vi "SUB_TimeGAP_SFCS_RTC.vi"(1 "SFCS year":i32, 2 "UUT_DateTime_input":string="20140703155955", 3 "SFCS month":i32, 4 "SFCS day":i32, 5 "SFCS hour":i32, 6 "SFCS minute":i32, 7 "SFCS second":i32) -> (0 "TimeGap(sec)":dbl format="%#_8f")   [LabVIEW 2011]
panel:
  out "current time":timestamp
  out "time stamp":timestamp
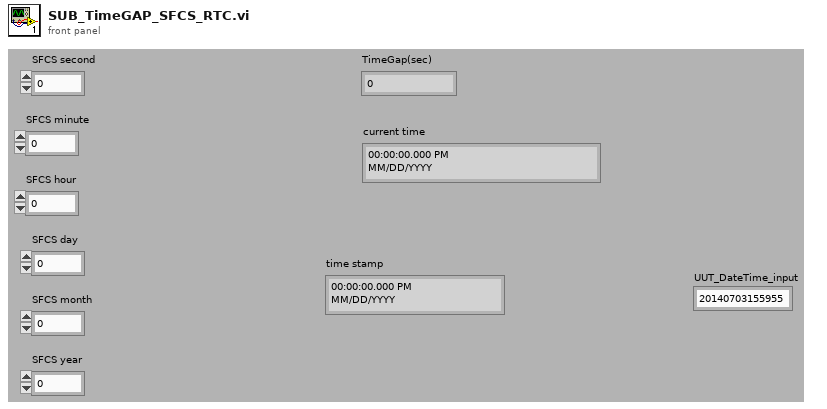
[diagram p1: front panel]
types:
  T1 = cluster{dbl, "SFCS second":i32, "SFCS minute":i32, "SFCS hour":i32, "SFCS day":i32, "SFCS month":i32, "SFCS year":i32, i32, i32, i32}
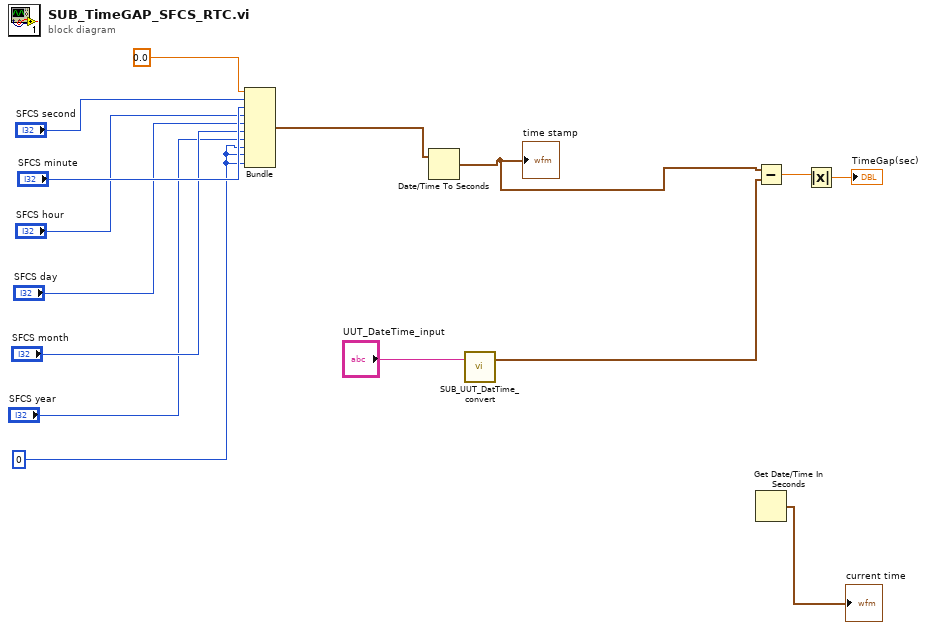
[diagram p0: block diagram]
diagram:
  w8 = 0
  n1 = Bundle(0.0, "SFCS second"="SFCS second", "SFCS minute"="SFCS minute", "SFCS hour"="SFCS hour", "SFCS day"="SFCS day", "SFCS month"="SFCS month", "SFCS year"="SFCS year", w8, w8, w8) -> (w7:T1)  [unwired: 1 in]
  n2 = Date/Time To Seconds(2:w7) -> (0:w6:timestamp)  [unwired: 1 in]
  "time stamp" <- w6
  n3 = call "SUB_UUT_DatTime_convert.vi"("UUT_DateTime_input"="UUT_DateTime_input") -> ("UUT TimeStamp out"=w2:timestamp)  [unwired: 2 in]
  n4 = Subtract(x=w6, y=w2) -> (x-y=w4:dbl)
  n5 = Get Date/Time In Seconds() -> (seconds since 1Jan1904=→"current time":timestamp)
  n6 = Absolute Value(x=w4) -> (abs(x)=→"TimeGap(sec)":dbl)
